vi "探头温度显示.vi"(11 "校准参数":u16(ring) caption="校准参数：" items=["pH", "DO", "浊度", "电导率", "叶绿素a", "藻密度", "ORP", "DO2"]) -> (3 "温度数据":sgl, 5 "温度偏移修正值":sgl)   [LabVIEW 2016, in "斯坦道多参数.lvlib"]
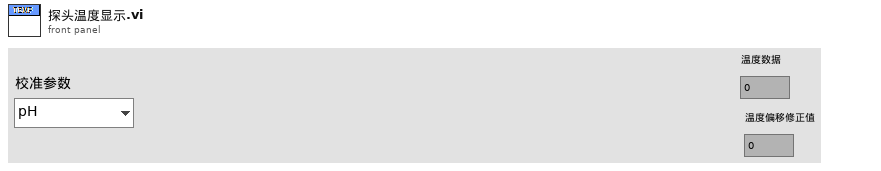
[diagram p1: front panel]
types:
  T1 = cluster{"pH探头选择":u16, "DO探头选择":u16, "电导率探头选择":u16, "浊度探头选择":u16, "叶绿素a探头选择":u16, "蓝绿藻探头选择":u16, "orp探头选择":u16, "COD探头选择":u16, "DO2探头选择":u16}
  T2 = cluster{"电极状态标志":u16, "电极型号标志":u16, "酸碱度测量值":sgl, "温度测量值":sgl, "酸碱度信号值":sgl, "温度信号值":sgl, "酸碱度偏移修正值":sgl, "温度偏移修正值":sgl, "手动温度补偿值":sgl, "酸碱度电极零点":sgl, "酸碱度电极斜率":sgl, "第1点标准值记录":sgl, "第1点信号值记录":sgl, "第1点温度值记录":sgl, "第2点标准值记录":sgl, "第2点信号值记录":sgl, "第2点温度值记录":sgl, "命令滤波设定":u16, "温度模式":enum16{"ATC", "MTC"}, "生产批次":u16, "电极序号":u16, "串口地址":u16, "串口波特率":enum16{"9600", "19200", "115200"}, "串口校验位":enum16{"NONE", "ODD", "EVEN"}, "串口停止位":enum16{"1bit", "2bit"}, "第一点标准值":sgl, "第二点标准值":sgl}
  T3 = cluster{"报警码":u16, "pH数值":sgl, "0X0003_NC":sgl, "温度数据":sgl, "pH原始信号 mv":sgl, "0X0009_NC":string, "产品名称":string, "序列号":string, "硬件版本":string, "软件版本":string, "通讯地址":u16, "波特率":u16, "设备类型":u16, "0X0026_NC":string, "第一点原始数据":sgl, "第一点校准数据":sgl, "第二点原始数据":sgl, "第二点校准数据":sgl, "探头校准命令":u16, "温度校准参数":sgl, "温度校准命令":u16}
  T4 = cluster{"电极状态标志":u16, "电极型号标志":u16, "溶解氧测量值":sgl, "温度测量值":sgl, "溶解氧饱和度值":sgl, "盐度补偿值":sgl, "大气压补偿值":sgl, "溶解氧偏移修正值":sgl, "温度偏移修正值":sgl, "手动温度补偿值":sgl, "溶解氧电极零点":sgl, "溶解氧电极斜率":sgl, "第1点标准值记录":sgl, "第1点信号值记录":sgl, "第1点温度值记录":sgl, "第2点标准值记录":sgl, "第2点信号值记录":sgl, "第2点温度值记录":sgl, "命令滤波设定":u16, "温度模式":enum16{"ATC", "MTC"}, "生产批次":u16, "电极序号":u16, "串口地址":u16, "串口波特率":enum16{"9600", "19200", "115200"}, "串口校验位":enum16{"NONE", "ODD", "EVEN"}, "串口停止位":enum16{"1bit", "2bit"}, "第一点标准值":sgl, "第二点标准值":sgl}
  T5 = cluster{"报警码":u16, "溶解氧数值（mg/L）":sgl, "溶解氧数据（%）":sgl, "温度数据":sgl, "溶解氧原始信号 nA":sgl, "大气压力":sgl, "盐度":sgl, "0X0009_NC":string, "产品名称":string, "序列号":string, "硬件版本":string, "软件版本":string, "通讯地址":u16, "波特率":u16, "设备类型":u16, "0X0026_NC":string, "第一点原始数据":sgl, "第一点校准数据":sgl, "第二点原始数据":sgl, "第二点校准数据":sgl, "探头校准命令":u16, "温度校准参数":sgl, "温度校准命令":u16}
  T6 = cluster{"电极状态标志":u16, "电极型号标志":u16, "浊度测量值":sgl, "温度测量值":sgl, "浊度信号值":sgl, "浊度偏移修正值":sgl, "温度偏移修正值":sgl, "手动温度补偿值":sgl, "浊度电极零点":sgl, "浊度电极斜率":sgl, "清洁周期":u16, "命令滤波设定":u16, "温度模式":enum16{"ATC", "MTC"}, "生产批次":u16, "电极序号":u16, "串口地址":u16, "串口波特率":enum16{"9600", "19200", "115200"}, "串口校验位":enum16{"NONE", "ODD", "EVEN"}, "串口停止位":enum16{"1bit", "2bit"}, "第一点标准值":sgl, "第二点标准值":sgl, "第三点标准值":sgl}
  T7 = cluster{"报警码":u16, "浊度数值 NTU":sgl, "温度数据":sgl, "原始光强数值":u16, "量程":u16, "平均次数":u16, "清扫模式":u16, "清扫次数":u16, "清扫间隔分钟":u16, "0X000B_NC":string, "产品名称":string, "序列号":string, "硬件版本":string, "软件版本":string, "通讯地址":u16, "波特率":u16, "设备类型":u16, "0X0026_NC":string, "校准量程":u16, "第一点原始光强":u16, "第一点校准数据":sgl, "第二点原始光强":u16, "第二点校准数据":sgl, "第三点原始光强":u16, "第三点校准数据":sgl, "探头校准命令":u16, "温度校准参数":sgl, "温度校准命令":u16}
  T8 = cluster{"电极状态标志":u16, "电极型号标志":u16, "电导率测量值":sgl, "温度测量值":sgl, "电导率信号值":sgl, "温度信号值":sgl, "温度补偿系数":sgl, "电导率偏移修正值":sgl, "温度偏移修正值":sgl, "手动温度补偿值":sgl, "电导率电极零点":sgl, "电导率电极斜率":sgl, "命令滤波设定":u16, "温度模式":enum16{"ATC", "MTC"}, "生产批次":u16, "电极序号":u16, "串口地址":u16, "串口波特率":enum16{"9600", "19200", "115200"}, "串口校验位":enum16{"NONE", "ODD", "EVEN"}, "串口停止位":enum16{"1bit", "2bit"}, "第一点标准值":sgl, "第二点标准值":sgl}
  T9 = cluster{"报警码":u16, "电导率数据（uS/cm）":sgl, "0x0003 NC":sgl, "温度数据":sgl, "电导率原始信号电阻":sgl, "当前量程":u16, "温度补偿系数":sgl, "0X0009_NC":string, "产品名称":string, "序列号":string, "硬件版本":string, "软件版本":string, "通讯地址":u16, "波特率":u16, "设备类型":u16, "0X0026_NC":string, "第一点原始数据":sgl, "第一点校准数据":sgl, "0X0035_NC":sgl, "0X0037_NC":sgl, "探头校准命令":u16, "温度校准参数":sgl, "温度校准命令":u16}
  T10 = cluster{"报警码":u16, "叶绿素a":sgl, "温度数据":sgl, "原始光强数值":u16, "量程":u16, "平均次数":u16, "清扫模式":u16, "清扫次数":u16, "清扫间隔分钟":u16, "0X000B_NC":string, "产品名称":string, "序列号":string, "硬件版本":string, "软件版本":string, "通讯地址":u16, "波特率":u16, "设备类型":u16, "0X0026_NC":string, "校准量程":u16, "第一点原始光强":u16, "第一点校准数据":sgl, "第二点原始光强":u16, "第二点校准数据":sgl, "第三点原始光强":u16, "第三点校准数据":sgl, "探头校准命令":u16, "温度校准参数":sgl, "温度校准命令":u16}
  T11 = cluster{"报警码":u16, "蓝绿藻":sgl, "温度数据":sgl, "原始光强数值":u16, "量程":u16, "平均次数":u16, "清扫模式":u16, "清扫次数":u16, "清扫间隔分钟":u16, "0X000B_NC":string, "产品名称":string, "序列号":string, "硬件版本":string, "软件版本":string, "通讯地址":u16, "波特率":u16, "设备类型":u16, "0X0026_NC":string, "校准量程":u16, "第一点原始光强":u16, "第一点校准数据":sgl, "第二点原始光强":u16, "第二点校准数据":sgl, "第三点原始光强":u16, "第三点校准数据":sgl, "探头校准命令":u16, "温度校准参数":sgl, "温度校准命令":u16}
  T12 = cluster{"电极状态标志":u16, "电极型号标志":u16, "测量值":sgl, "温度测量值":sgl, "信号值":sgl, "温度信号值":sgl, "000AH_NC":sgl, "偏移修正值":sgl, "温度偏移修正值":sgl, "手动温度补偿值":sgl, "命令滤波设定":u16, "温度模式":enum16{"ATC", "MTC"}, "生产批次":u16, "传感器序号":u16, "串口地址":u16, "串口波特率":enum16{"9600", "19200", "115200"}, "串口校验位":enum16{"NONE", "ODD", "EVEN"}, "串口停止位":enum16{"1bit", "2bit"}}
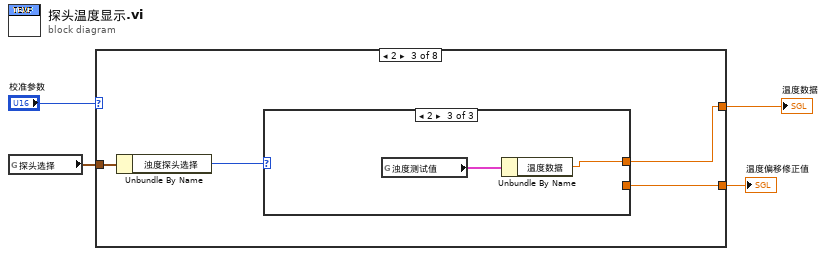
[diagram p0: block diagram]
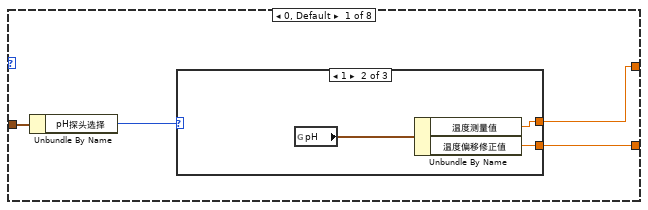
[diagram p2: hidden frame]
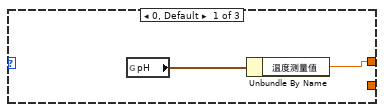
[diagram p3: hidden frame]
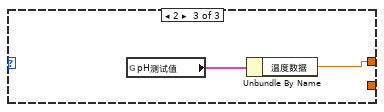
[diagram p4: hidden frame]
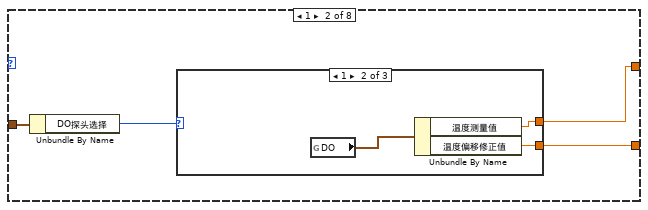
[diagram p5: hidden frame]
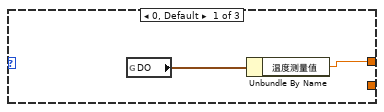
[diagram p6: hidden frame]
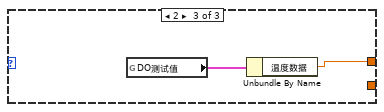
[diagram p7: hidden frame]
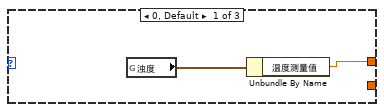
[diagram p8: hidden frame]
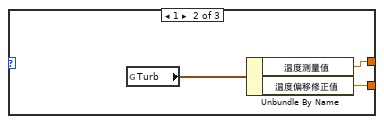
[diagram p9: hidden frame]
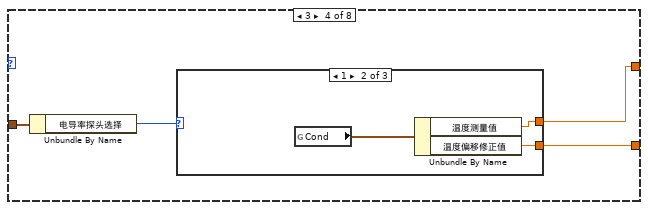
[diagram p10: hidden frame]
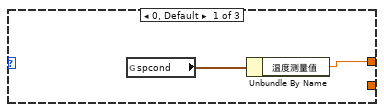
[diagram p11: hidden frame]
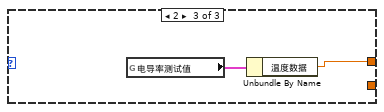
[diagram p12: hidden frame]
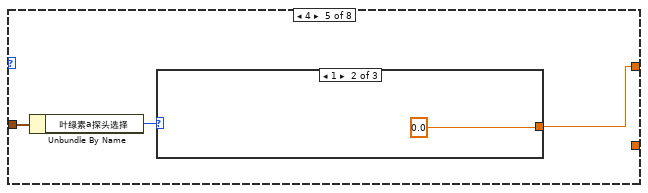
[diagram p13: hidden frame]
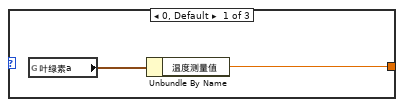
[diagram p14: hidden frame]
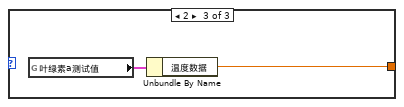
[diagram p15: hidden frame]
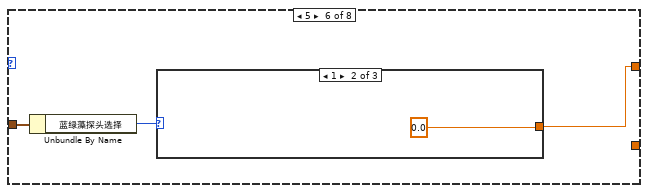
[diagram p16: hidden frame]
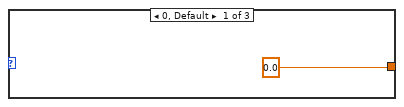
[diagram p17: hidden frame]
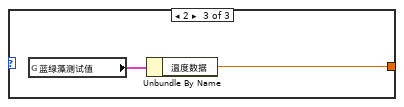
[diagram p18: hidden frame]
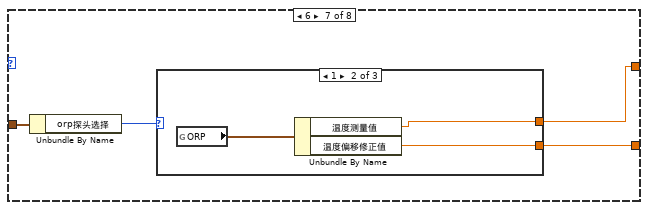
[diagram p19: hidden frame]
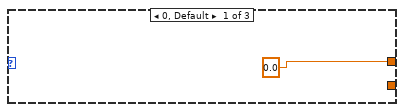
[diagram p20: hidden frame]
diagram:
  n1 = global read "断电保存变量.vi" "探头选择"() -> (w2:T1)
  n2 = case shown="2" "校准参数" {
    tunnel: [w7 w18 w29 w40 w50 w58 w66 w74] -> w4
    tunnel: w2 -> [w6 w17 w28 w39 w49 w57 w65 _]
    tunnel: [w5 w16 w27 w38 _ _ w64 _] -> w1
    frame 0, Default {
      n3 = Unbundle By Name(w6) -> ("pH探头选择"=w8:u16)
      n4 = case shown="1" w8 {
        tunnel: [w9 w12 w15] -> w7
        tunnel: [_ w11 _] -> w5
        frame 0, Default {
          n5 = global read "禹山过程全局变量.vi" "pH"() -> (w10:cluster{"温度测量值":sgl, "ORP":sgl, "pH":sgl})
          n6 = Unbundle By Name(w10) -> ("温度测量值"=w9:sgl)
        }
        frame 1 {
          n7 = global read "国弘过程全局变量.vi" "pH"() -> (w13:T2)
          n8 = Unbundle By Name(w13) -> ("温度测量值"=w12:sgl, "温度偏移修正值"=w11:sgl)
        }
        frame 2 {
          n9 = global read "纳清过程全局变量.vi" "pH测试值"() -> (w14:T3)
          n10 = Unbundle By Name(w14) -> ("温度数据"=w15:sgl)
        }
      }
    }
    frame 1 {
      n11 = Unbundle By Name(w17) -> ("DO探头选择"=w19:u16)
      n12 = case shown="1" w19 {
        tunnel: [w20 w23 w26] -> w18
        tunnel: [_ w22 _] -> w16
        frame 0, Default {
          n13 = global read "禹山过程全局变量.vi" "DO"() -> (w21:cluster{"温度测量值":sgl, "DO%":sgl, "DOmg/L":sgl})
          n14 = Unbundle By Name(w21) -> ("温度测量值"=w20:sgl)
        }
        frame 1 {
          n15 = global read "国弘过程全局变量.vi" "DO"() -> (w24:T4)
          n16 = Unbundle By Name(w24) -> ("温度测量值"=w23:sgl, "温度偏移修正值"=w22:sgl)
        }
        frame 2 {
          n17 = global read "纳清过程全局变量.vi" "DO测试值"() -> (w25:T5)
          n18 = Unbundle By Name(w25) -> ("温度数据"=w26:sgl)
        }
      }
    }
    frame 2 {
      n19 = Unbundle By Name(w28) -> ("浊度探头选择"=w30:u16)
      n20 = case shown="2" w30 {
        tunnel: [w31 w34 w37] -> w29
        tunnel: [_ w33 _] -> w27
        frame 0, Default {
          n21 = global read "禹山过程全局变量.vi" "浊度"() -> (w32:cluster{"温度测量值":sgl, "浊度测量值":sgl})
          n22 = Unbundle By Name(w32) -> ("温度测量值"=w31:sgl)
        }
        frame 1 {
          n23 = global read "国弘过程全局变量.vi" "Turb"() -> (w35:T6)
          n24 = Unbundle By Name(w35) -> ("温度测量值"=w34:sgl, "温度偏移修正值"=w33:sgl)
        }
        frame 2 {
          n25 = global read "纳清过程全局变量.vi" "浊度测试值"() -> (w36:T7)
          n26 = Unbundle By Name(w36) -> ("温度数据"=w37:sgl)
        }
      }
    }
    frame 3 {
      n27 = Unbundle By Name(w39) -> ("电导率探头选择"=w41:u16)
      n28 = case shown="1" w41 {
        tunnel: [w42 w45 w48] -> w40
        tunnel: [_ w44 _] -> w38
        frame 0, Default {
          n29 = global read "禹山过程全局变量.vi" "spcond"() -> (w43:cluster{"温度测量值":sgl, "测量值":sgl, "错误标志":u16})
          n30 = Unbundle By Name(w43) -> ("温度测量值"=w42:sgl)
        }
        frame 1 {
          n31 = global read "国弘过程全局变量.vi" "Cond"() -> (w46:T8)
          n32 = Unbundle By Name(w46) -> ("温度测量值"=w45:sgl, "温度偏移修正值"=w44:sgl)
        }
        frame 2 {
          n33 = global read "纳清过程全局变量.vi" "电导率测试值"() -> (w47:T9)
          n34 = Unbundle By Name(w47) -> ("温度数据"=w48:sgl)
        }
      }
    }
    frame 4 {
      n35 = Unbundle By Name(w49) -> ("叶绿素a探头选择"=w51:u16)
      n36 = case shown="1" w51 {
        tunnel: [w52 sgl 0.0 ("温度数据") w56] -> w50
        frame 0, Default {
          n37 = global read "禹山过程全局变量.vi" "叶绿素a"() -> (w53:cluster{"温度测量值":sgl, "叶绿素测量值":sgl, "错误标志":u16})
          n38 = Unbundle By Name(w53) -> ("温度测量值"=w52:sgl)
        }
        frame 1 {
        }
        frame 2 {
          n39 = global read "纳清过程全局变量.vi" "叶绿素a测试值"() -> (w55:T10)
          n40 = Unbundle By Name(w55) -> ("温度数据"=w56:sgl)
        }
      }
    }
    frame 5 {
      n41 = Unbundle By Name(w57) -> ("蓝绿藻探头选择"=w59:u16)
      n42 = case shown="1" w59 {
        tunnel: [sgl 0.0 ("温度数据") sgl 0.0 ("温度数据") w63] -> w58
        frame 0, Default {
        }
        frame 1 {
        }
        frame 2 {
          n43 = global read "纳清过程全局变量.vi" "蓝绿藻测试值"() -> (w62:T11)
          n44 = Unbundle By Name(w62) -> ("温度数据"=w63:sgl)
        }
      }
    }
    frame 6 {
      n45 = Unbundle By Name(w65) -> ("orp探头选择"=w67:u16)
      n46 = case shown="1" w67 {
        tunnel: [sgl 0.0 ("温度数据") w70 sgl 0.0 ("温度测量值")] -> w66
        tunnel: [_ w69 _] -> w64
        frame 0, Default {
        }
        frame 1 {
          n47 = global read "国弘过程全局变量.vi" "ORP"() -> (w71:T12)
          n48 = Unbundle By Name(w71) -> ("温度测量值"=w70:sgl, "温度偏移修正值"=w69:sgl)
        }
        frame 2 {
        }
      }
    }
    frame 7 {
      n49 = global read "禹山过程全局变量.vi" "DO 2"() -> (w73:cluster{"温度测量值":sgl, "DO%":sgl, "DOmg/L":sgl})
      n50 = Unbundle By Name(w73) -> ("温度测量值"=w74:sgl)
    }
  }
  "温度数据" <- w4
  "温度偏移修正值" <- w1
